vi "NF87XX.constructor.vi"(0 "name":string, 2 "data in":string, 5 "error in(no error)":errorcluster) -> (14 "i ref out":refnum<vi>, 16 "data out":string, 19 "error out":errorcluster)   [LabVIEW 2014, in "NF87XX.lvlib"]
doc: "This class controls an \"Intelligent Picomoter Driver\" 8753 from New Focus. The communication is performed via the \"Picomoter Ethernet Controller\" 8752 from New Focus which is connected to a computer via RS232 or using the ethernet (TCP(IP). Up to 32 drivers 8743 can be connected to one controller 8752. Each driver operates one mirror adjuster. Each mirror adjuster has three axes driven by piezo motors.\n\nThis class uses an instrument driver which bases on \"Example_LabVIEW 6.1_MCL Rev E\" which can be downloaded from New Focus. This driver had to be totally renewed to operate properly.\n\nauthor: Stefan Götte, GSI\ndata: 30-AUG-2006\n\nLicense Agreement for this software:\n\nCopyright (C)\nGesellschaft für Schwerionenforschung, GSI\nPlanckstr. 1\n64291 Darmstadt\nGermany\n\nContact: D.Beck@gsi.de \n\nThis program is free software; you can redistribute it and/or modify it under the terms of the \nGNU General Public License as published by the Free Software Foundation; either version 2 of \nthe license, or (at your option) any later version.\n\nThis program is distributed in the hope that it will be useful, but WITHOUT ANY WARRANTY; \nwithout even the implied warranty of MERCHANTABILITY or FITNESS FOR A PARTICULAR PURPOSE. See the GNU General License for more details (http://www.gnu.org).\n\nGesellschaft für Schwerionenforschung, GSI\nPlanckstr. 1, 64291 Darmstadt, Germany\nFor all questions and ideas contact: M.Richter@gsi.de, H.Brand@gsi.de or D.Beck@gsi.de.\nLast update: 16-JUN-2004"
uses:
  NF87XX.lvlib
  NF87XX.driver Type.ctl
  CS_Core/BaseProcess/BaseProcess.lvlib
  CS_Core/CSSystem/CSSystemLib/CSSystemLib.lvlib
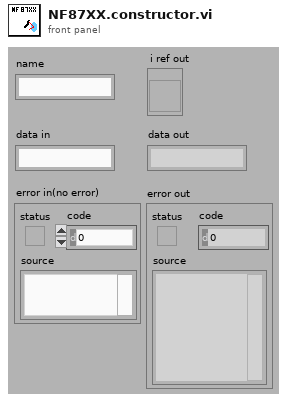
[diagram p1: front panel]
types:
  T1 = enum16{"SetAttribute", "GetAttribute", "CreateAttribute", "DestroyAttribute", "DestroyAllAtributes"}
  T2 = enum16{"simple", "synchronous", "asynchronous", "notification"}
  T3 = typedef "NF87XX.lvlib/NF87XX.driver Type.ctl" = enum16{"not defined", "3-ch open loop drv", "1-ch closed loop drv"}
  T4 = typedef "NF87XX.lvlib/NF87XX.i attribute.ctl" = cluster{"Con Settings":T5, "Drivers":T6[], "Status":cluster{"Service ID":i32, "Status":T8}, "Joystick available":bool, "VISA Resource":string}
  T5 = typedef "NewFocusPico - Driver np.lvlib/VISA & TCPIP Control.ctl" = cluster{"VISA or TCP/IP":bool, "Init Connection":bool, "Close Connection":bool, "Resource Name":refnum<visa-resource-name>, "hostname":string, "connection ID":refnum<k5>}
  T6 = typedef "NF87XX.lvlib/NF87XX.driver Settings.ctl" = cluster{"Name":string, "Driver Type":T3, "Pico Parameter type":T7, "Acceleration [Steps/s²]":cluster{"Motor 0":dbl, "Motor 1":dbl, "Motor 2":dbl}, "Start Velocity [Steps/s]":cluster{"Motor 0":dbl, "Motor 1":dbl, "Motor 2":dbl}, "Velocity [Steps/s]":cluster{"Motor 0":dbl, "Motor 1":dbl, "Motor 2":dbl}, "axis channel":i32, "Position":i32, "Position Service ID":i32}
  T7 = typedef "NewFocusPico - Driver np.lvlib/Pico Parameters.ctl" = cluster{"Pico Type":enum16{"Open-Loop Pico", "Close-Loop Pico", "Pico Ultra"}, "Acceleration (steps/sec^2)":string, "Velocity ( Hz)":string, "Driver":string, "Motor":string, "Channel":string, "Process Step":string}
  T8 = typedef "PH_StatusHandler.lvlib/PH_StatusHandler.Status.ctl" = i16
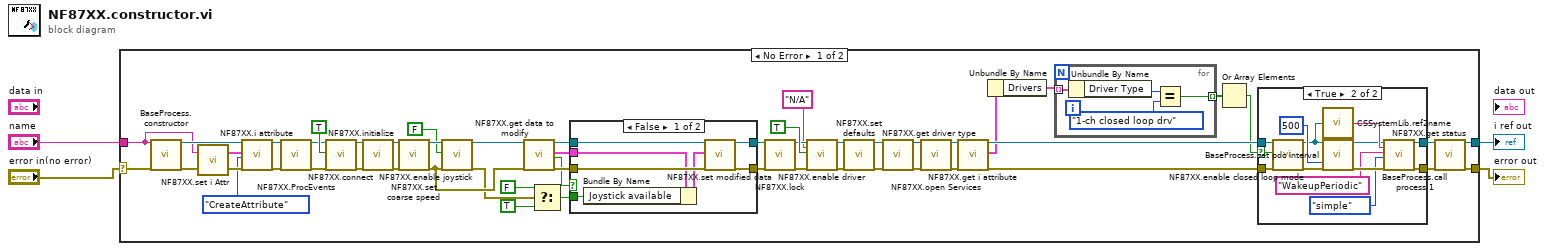
[diagram p0: block diagram]
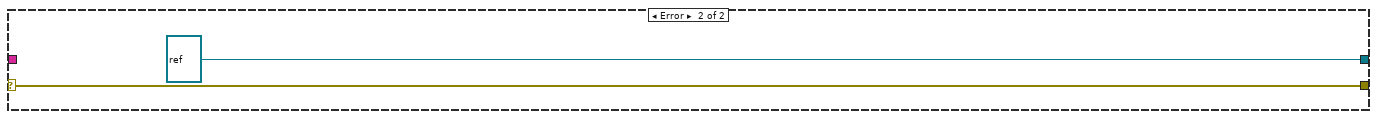
[diagram p4: hidden frame]
diagram:
  n1 = case shown="No Error" "error in(no error)" {
    selector: "error in(no error)" -> [w48 w86]
    tunnel: "name" -> [w7 _]
    tunnel: [w45 w86] -> w3
    tunnel: [w46 refnum<vi> refnum ("i ref out")] -> w2
    frame No Error {
      n2 = call "BaseProcess.constructor.vi"("name"=w7, "error in (no error)"=w48) -> ("i ref out"=w56:refnum<vi>, "error out"=w9:errorcluster)  [unwired: 15 in, 1 out]
      n3 = call "NF87XX.set i Attr.vi"("error in (no error)"=w9, "DB Entry to read"=w7) -> ("error out"=w8:errorcluster, "i Attributes"=w6:T4)
      n4 = call "NF87XX.i attribute.vi"("VI Refnum"=w56, "CLASS.i attribute"=w6, "Action"=T1."CreateAttribute", "error in (no error)"=w8) -> ("VI Refnum out"=w55:refnum<vi>, "error out"=w54:errorcluster)  [unwired: 13 in, 1 out]
      n5 = call "NF87XX.ProcEvents.vi"("i ref in"=w55, "error in"=w54) -> ("i ref out"=w11:refnum<vi>, "error out"=w10:errorcluster)  [unwired: 16 in]
      n6 = call "NF87XX.connect.vi"("i ref in"=w11, "Connect?"=TRUE ("Open VISA?"), "error in (no error)"=w10) -> ("i ref out"=w49:refnum<vi>, "error out"=w24:errorcluster)  [unwired: 15 in]
      n7 = call "NF87XX.initialize.vi"("i ref in"=w49, "error in (no error)"=w24) -> ("i ref out"=w27:refnum<vi>, "error out"=w26:errorcluster)  [unwired: 16 in]
      n8 = call "NF87XX.set coarse speed.vi"("i ref in"=w27, "error in (no error)"=w26) -> ("i ref out"=w28:refnum<vi>, "error out"=w23:errorcluster)  [unwired: 16 in]
      n9 = call "NF87XX.enable joystick.vi"("i ref in"=w28, "Enable Joystick"=FALSE, "error in (no error)"=w23) -> ("i ref out"=w22:refnum<vi>, "error out"=w15:errorcluster)  [unwired: 15 in]
      n10 = call "NF87XX.get data to modify.vi"("i ref in"=w22, "error in (no error)"=w23) -> ("i ref out"=w20:refnum<vi>, "i attribute"=w16:T4, "timed out"=w17:bool, "error out"=w21:errorcluster)  [unwired: 14 in]
      n11 = Select(t=FALSE ("Enable Joystick"), s=w15, f=TRUE) -> (s? t:f=w12:bool)
      n12 = case shown="False" w17 {
        tunnel: w21 -> [w63 w64]
        tunnel: w20 -> [w62 w65]
        tunnel: [w61 w65] -> w19
        tunnel: [w60 w64] -> w18
        tunnel: w16 -> [w59 _]
        tunnel: w12 -> [w57 _]
        frame False {
          n13 = Bundle By Name(cluster=w59, "Joystick available"=w57) -> (w58:T4)
          n14 = call "NF87XX.set modified data.vi"("i ref in"=w62, "i attribute"=w58, "error in (no error)"=w63) -> ("i ref out"=w61:refnum<vi>, "error out"=w60:errorcluster)  [unwired: 15 in]
        }
        frame True {
        }
      }
      n15 = call "NF87XX.lock.vi"("i ref in"=w19, "error in (no error)"=w18) -> ("i ref out"=w51:refnum<vi>, "error out"=w52:errorcluster)  [unwired: 16 in]
      n16 = call "NF87XX.enable driver.vi"("i ref in"=w51, "System"="N/A", "Enable Driver"=TRUE, "error in (no error)"=w52) -> ("i ref out"=w37:refnum<vi>, "error out"=w36:errorcluster)  [unwired: 14 in]
      n17 = call "NF87XX.set defaults.vi"("i ref in"=w37, "error in (no error)"=w36) -> ("i ref out"=w43:refnum<vi>, "error out"=w44:errorcluster)  [unwired: 16 in]
      n18 = call "NF87XX.get driver type.vi"("i ref in"=w43, "error in (no error)"=w44) -> ("i ref out"=w32:refnum<vi>, "error out"=w30:errorcluster)  [unwired: 15 in, 1 out]
      n19 = call "NF87XX.open Services.vi"("i ref in"=w32, "error in (no error)"=w30) -> ("i ref out"=w31:refnum<vi>, "error out"=w29:errorcluster)  [unwired: 16 in]
      n20 = call "NF87XX.get i attribute.vi"("i ref in"=w31, "error in (no error)"=w29) -> ("i ref out"=w41:refnum<vi>, "i attribute"=w40:T4, "error out"=w42:errorcluster)  [unwired: 15 in]
      n21 = Unbundle By Name(w40) -> ("Drivers"=w39:T6[])
      n22 = for {
        tunnel: w39 -> [w84] mode=indexing
        tunnel: [w81] -> w38 mode=indexing
        n23 = Unbundle By Name(w84) -> ("Driver Type"=w83:T3)
        n24 = Equal?(x=w83, y=NF87XX.driver_Type."1-ch closed loop drv") -> (x = y?=w81:bool)
      }
      n25 = Or Array Elements(Boolean array=w38) -> (logical OR=w35:bool)
      n26 = case shown="True" w35 {
        selector: w35 -> [_ w78]
        tunnel: [w67 w73] -> w33
        tunnel: [w66 w72] -> w34
        tunnel: w42 -> [w67 w80]
        tunnel: w41 -> [w66 w79]
        frame False {
        }
        frame True {
          n27 = call "NF87XX.enable closed loop mode.vi"("i ref in"=w79, "Enable closed loop mode"=w78, "error in (no error)"=w80) -> ("i ref out"=w69:refnum<vi>, "error out"=w71:errorcluster)  [unwired: 15 in]
          n28 = call "CSSystemLib.ref2name.vi"("obj refnum"=w69) -> ("name"=w75:string)
          n29 = call "BaseProcess.set pdc interval.vi"("i ref in"=w69, "PeriodicInterval [ms]"=500 ("PeriodicInterval"), "error in (no error)"=w71) -> ("i ref out"=w68:refnum<vi>, "error out"=w77:errorcluster)  [unwired: 14 in, 1 out]
          n30 = call "BaseProcess.call process 1.vi"("i ref in"=w68, "Object"=w75, "Selector"="WakeupPeriodic", "CallType"=T2."simple", "error in (no error)"=w77) -> ("i ref out"=w72:refnum<vi>, "error out"=w73:errorcluster)  [unwired: 12 in, 1 out]
        }
      }
      n31 = call "NF87XX.get status.vi"("i ref in"=w34, "error in (no error)"=w33) -> ("i ref out"=w46:refnum<vi>, "error out"=w45:errorcluster)  [unwired: 15 in, 1 out]
    }
    frame Error {
    }
  }
  "i ref out" <- w2
  "error out" <- w3
